vi "Clusterwitharrayextended.vi"(1 "Cluster In":cluster{"Array In":ext[], "Numeric Input":ext} {"Numeric Input" format="%.2f"; "Array In" format="%.2f"}, 2 "Base":ext format="%.2f") -> (0 "Cluster Out":cluster{"Array Out":ext[], "Numeric Output":ext} {"Numeric Output" format="%.2f"; "Array Out" format="%.2f"})   [LabVIEW 2011]
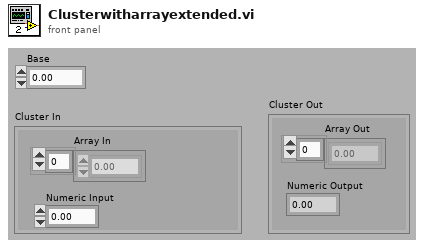
[diagram p1: front panel]
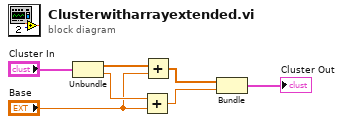
[diagram p0: block diagram]
diagram:
  n1 = Unbundle("Cluster In") -> ("Array In"=w7:ext[], "Numeric Input"=w6:ext)
  n2 = Add(x=w6, y="Base") -> (x+y=w4:ext)
  n3 = Add(x=w7, y="Base") -> (x+y=w5:ext[])
  n4 = Bundle(w5, w4) -> (→"Cluster Out":cluster{ext[], ext})  [unwired: 1 out]
